vi "CloseDevice.vi"(8 "error in (no error)":errorcluster, 11 "Acq Thread Data in":T1) -> (0 "error out":errorcluster, 3 "Acq Thread Data out":T1)   [LabVIEW 2019]
uses:
  Typedefs/Acquisition Thread/#cluster_AcqThreadData.ctl
  <vilib>/MagicBox/Device/Arduino/Arduino.lvclass
  <vilib>/MagicBox/Peripherals/POX/POX.lvclass
  Typedefs/Acquisition Thread/#enum_AcqThreadState.ctl
  Typedefs/#cluster_GUIRefs.ctl
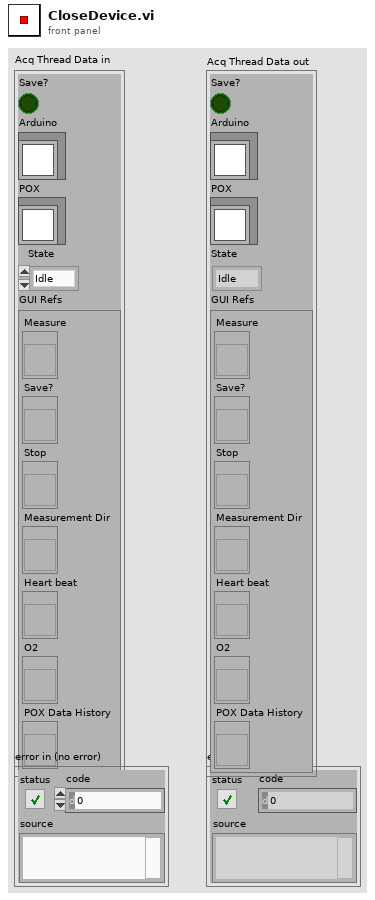
[diagram p1: front panel]
types:
  T1 = typedef "#cluster_AcqThreadData.ctl" = cluster{"Save?":bool, "Arduino":refnum<class "Arduino.lvclass">, "POX":refnum<class "POX.lvclass">, "State":T2, "GUI Refs":T3}
  T2 = typedef "#enum_AcqThreadState.ctl" = enum16{"Idle", "Operate", "Error"}
  T3 = typedef "#cluster_GUIRefs.ctl" = cluster{"Measure":refnum<vi>, "Save?":refnum<vi>, "Stop":refnum<vi>, "Measurement Dir":refnum<vi>, "Heart beat":refnum<vi>, "O2":refnum<vi>, "POX Data History":refnum<vi>}
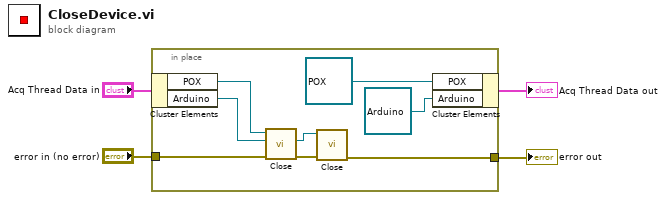
[diagram p0: block diagram]
diagram:
  n1 = in-place {
    in-place-border: "error in (no error)" -> [w12]
    in-place-border: [w5] -> w1
    n2 = in-place-cluster #1("Acq Thread Data in") -> ("POX"=w11:refnum<class "POX.lvclass">, "Arduino"=w10:refnum<class "Arduino.lvclass">)
    n3 = call-dynamic "Close.vi"("error in (no error)"=w12, "Arduino in"=w10, "POX in"=w11) -> ("error out"=w9:errorcluster, "Arduino out"=w8:refnum<class "Arduino.lvclass">)  [unwired: 6 in, 1 out]
    n4 = call-dynamic "Close.vi"("error in (no error)"=w9, "Arduino in"=w8) -> ("error out"=w5:errorcluster)  [unwired: 8 in, 1 out]
    n5 = in-place-cluster #1("POX"=refnum<class "POX.lvclass"> refnum, "Arduino"=refnum<class "Arduino.lvclass"> refnum) -> (→"Acq Thread Data out":T1)
  }
  "error out" <- w1
